vi "Kinect Extract Background.vi"() -> ()   [LabVIEW 2011]
uses:
  <vilib>/vision/Image Controls.llb/IMAQ Image.ctl
  <vilib>/vision/NI_Vision_Development_Module.lvlib
panel:
  in  "Morph Op":T1(ring)=enum."Open"
  in  "Post Proc Bounds 2":cluster{dbl, dbl}(slide)={0.0, 32768.0} scale=-3000.0..3000.0
  in  "Background Image In 2":T2
  out "Processed Image Out 2":T2
  out "error out 2":errorcluster
  in  "Post Proc Filter Divisor 2":sgl=1.0 min=0 max=1 step=0.1
  in  "Postproc Filter Size 2":i32 min=0 max=7
  in  "Divisor 2":sgl=1.0 min=0 max=1 step=0.1
  in  "Median Filter Size 2":i32 min=0 max=7
  in  "Distance to Camera Visible 2":cluster{dbl, dbl}(slide)={0.0, 32768.0} scale=-32768.0..32768.0
  in  "error in (no error) 2":errorcluster
  in  "Depth Image In 2":T2
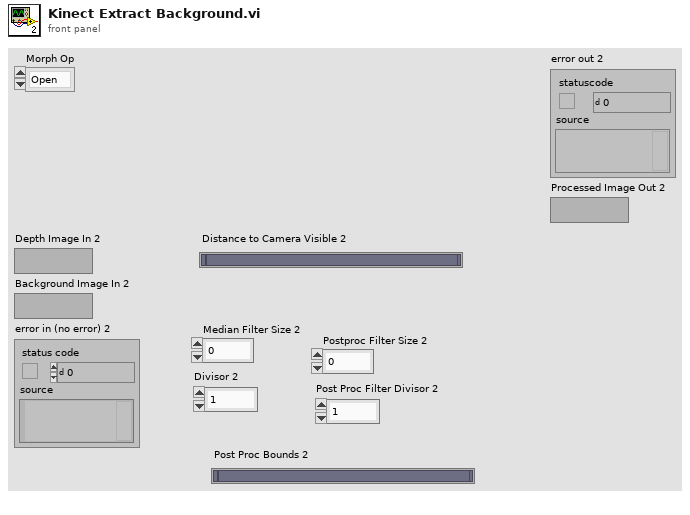
[diagram p1: front panel]
types:
  T1 = enum32{"AutoM", "Close", "Dilate", "Erode", "Gradient", "Gradient in", "Gradient out", "HitMiss", "Open", "PClose", "POpen", "Thick", "Thin"}
  T2 = typedef "IMAQ Image.ctl" = refnum<image>
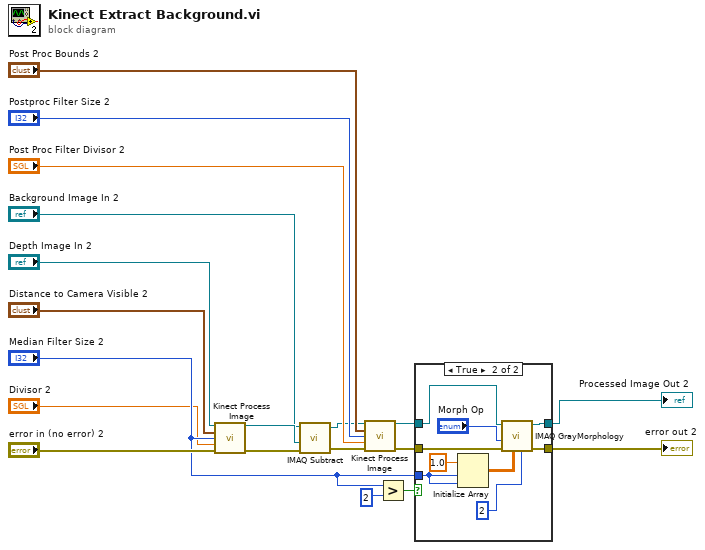
[diagram p0: block diagram]
diagram:
  n1 = call "Kinect Process Image.vi"("Depth Image In"="Depth Image In 2", "Distance to Camera Visible"="Distance to Camera Visible 2", "Median Filter Size"="Median Filter Size 2", "Divisor"="Divisor 2", "error in (no error)"="error in (no error) 2") -> ("Image Dst Out"=w15:T2, "error out"=w1:errorcluster)  [unwired: 9 in]
  n2 = call "IMAQ Subtract"("Image Src A"="Background Image In 2", "Image Src B"=w15, "error in (no error)"=w1) -> ("Image Dst Out"=w2:T2, "error out"=w7:errorcluster)  [unwired: 4 in]
  n3 = call "Kinect Process Image.vi"("Depth Image In"=w2, "Distance to Camera Visible"="Post Proc Bounds 2", "Median Filter Size"="Postproc Filter Size 2", "Divisor"="Post Proc Filter Divisor 2", "error in (no error)"=w7) -> ("Image Dst Out"=w6:T2, "error out"=w5:errorcluster)  [unwired: 9 in]
  n4 = Greater?(x="Median Filter Size 2", y=2) -> (0:w3:bool)
  n5 = case shown="True" w3 {
    tunnel: w6 -> [w20 w29]
    tunnel: w5 -> [w21 w28]
    tunnel: [w21 w27] -> w12
    tunnel: [w20 w26] -> w11
    tunnel: "Median Filter Size 2" -> [_ w23]
    frame False {
    }
    frame True {
      n6 = Initialize Array(1.0 ("element"), w23, w23) -> (w22:dbl[][])
      n7 = call "IMAQ GrayMorphology"("Number of iterations (1)"=2, "Structuring Element"=w22, "error in (no error)"=w28, "Operation"="Morph Op", "Image Src"=w29) -> ("error out"=w27:errorcluster, "Image Dst Out"=w26:T2)  [unwired: 5 in]
    }
  }
  "error out 2" <- w12
  "Processed Image Out 2" <- w11
